vi "kD2ATar.vi"(10 "Input":i16[](array[numeric])=[0, 0, 0, 0, 0, 0, 0, 0, 0, 0, 0, 0, 0, 0, 0, 0]) -> (2 "ToFIFO":u16[](array[numeric]))   [LabVIEW 2010, in "kevLib2011.lvlib"]
uses:
  kevLib2011.lvlib
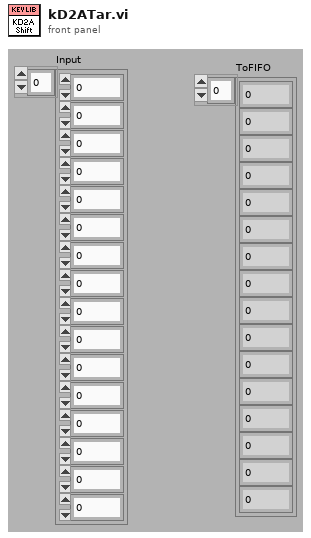
[diagram p1: front panel]
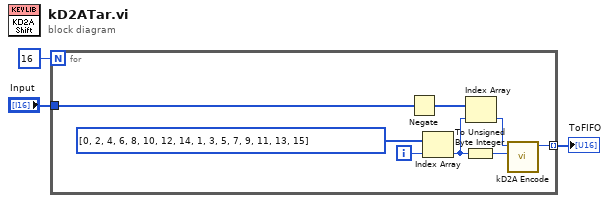
[diagram p0: block diagram]
diagram:
  n1 = for {
    N: 16 -> [_]
    tunnel: "Input" -> [w11]
    tunnel: [w7] -> w1 mode=indexing
    i -> [w9]
    n2 = Negate(x=w11) -> (-x=w4:i16[])
    n3 = Index Array(array=i32[] [0, 2, 4, 6, 8, 10, 12, 14, 1, 3, 5, 7, 9, 11, 13, 15], index=w9) -> (element=w5:i32)
    n4 = To Unsigned Byte Integer(number=w5) -> (unsigned 8bit integer=w6:u8)
    n5 = Index Array(array=w4, index=w5) -> (element=w8:i16)
    n6 = call "kD2A Encode.vi"("Position"=w6, "Value"=w8) -> ("Coded Output"=w7:u16)  [unwired: 9 in]
  }
  "ToFIFO" <- w1
